vi "isPrimitiveType.vi"(1 "field type":string) -> (0 "Boolean":bool)   [LabVIEW 2012]
doc: "Checks whether a type is a primative"
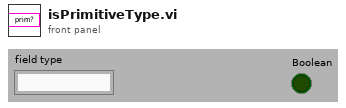
[diagram p1: front panel]
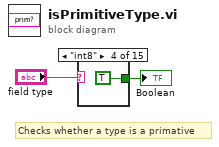
[diagram p0: block diagram]
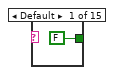
[diagram p2: hidden frame]
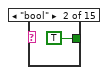
[diagram p3: hidden frame]
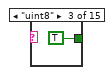
[diagram p4: hidden frame]
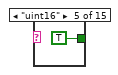
[diagram p5: hidden frame]
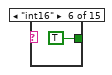
[diagram p6: hidden frame]
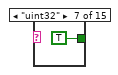
[diagram p7: hidden frame]
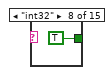
[diagram p8: hidden frame]
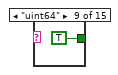
[diagram p9: hidden frame]
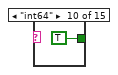
[diagram p10: hidden frame]
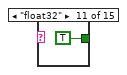
[diagram p11: hidden frame]
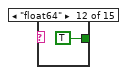
[diagram p12: hidden frame]
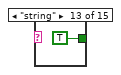
[diagram p13: hidden frame]
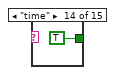
[diagram p14: hidden frame]
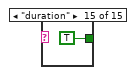
[diagram p15: hidden frame]
diagram:
  # "Checks whether a type is a primative"
  n1 = case shown="\"int8\"" "field type" {
    tunnel: [FALSE TRUE TRUE TRUE TRUE TRUE TRUE TRUE TRUE TRUE TRUE TRUE TRUE TRUE TRUE] -> w1
    frame Default {
    }
    frame "bool" {
    }
    frame "uint8" {
    }
    frame "int8" {
    }
    frame "uint16" {
    }
    frame "int16" {
    }
    frame "uint32" {
    }
    frame "int32" {
    }
    frame "uint64" {
    }
    frame "int64" {
    }
    frame "float32" {
    }
    frame "float64" {
    }
    frame "string" {
    }
    frame "time" {
    }
    frame "duration" {
    }
  }
  "Boolean" <- w1
